vi "11_LaserowaTransmisjaSzeregowaTypuSimplex.vi"() -> ()   [LabVIEW 2017]
uses:
  <vilib>/Instr/_visa.llb/VISA Configure Serial Port (Instr).vi
panel:
  in  "VISA resource name":refnum<visa-resource-name>
  in  "Zakończ":bool
  in  "Wyślij":bool
  in  "Tekst do wysłania":string
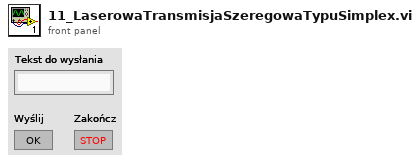
[diagram p1: front panel]
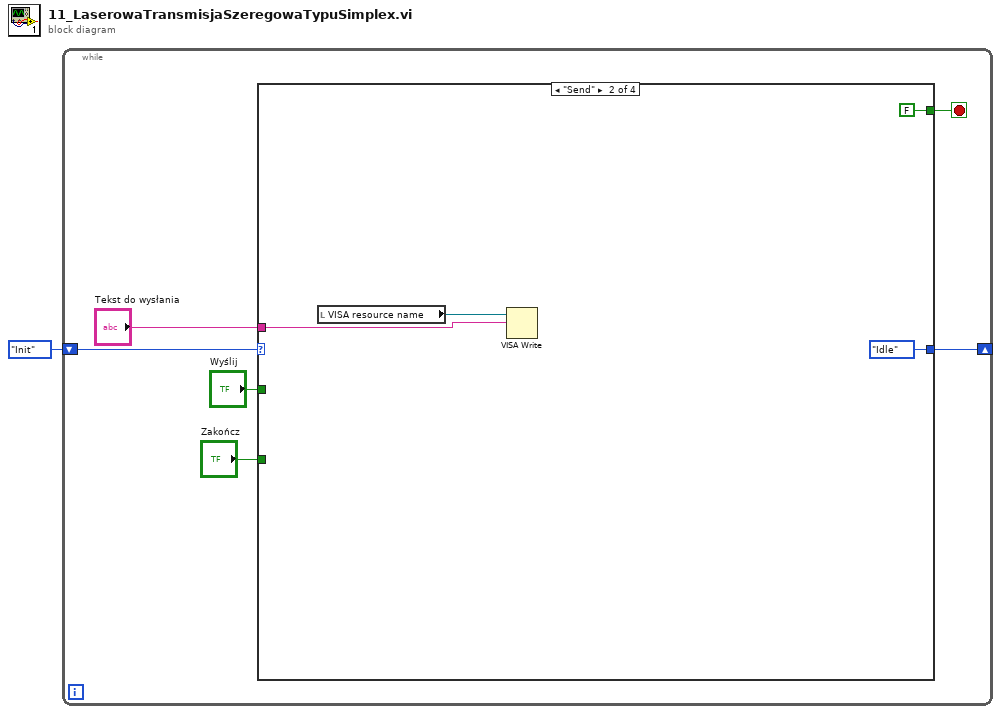
[diagram p0: block diagram]
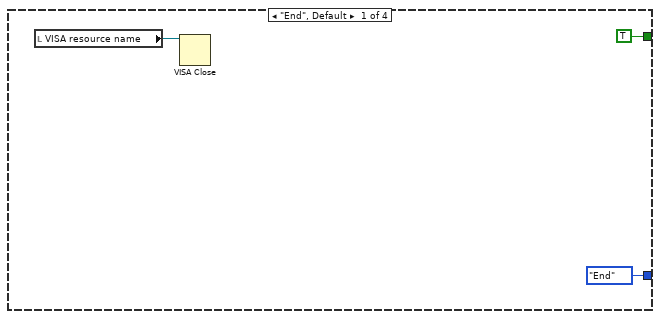
[diagram p2: hidden frame]
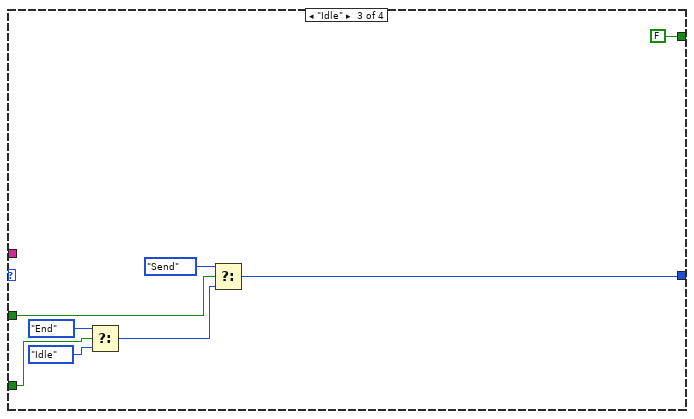
[diagram p3: hidden frame]
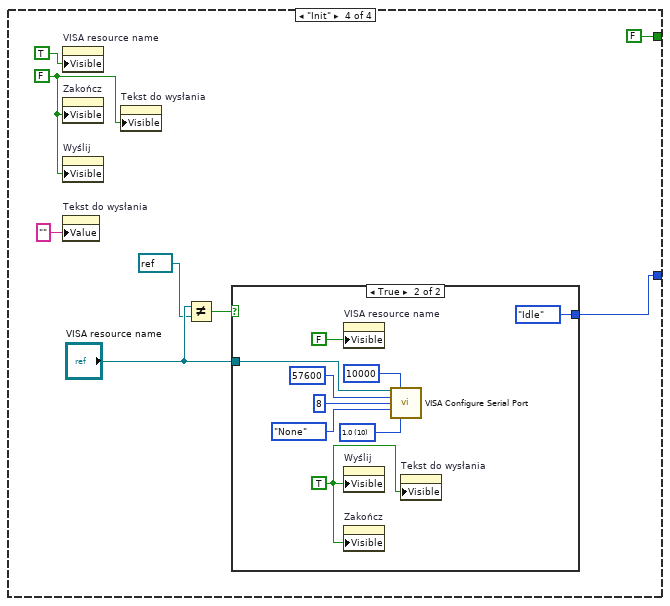
[diagram p4: hidden frame]
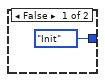
[diagram p5: hidden frame]
diagram:
  n1 = while {
    shift-right: [w3] -> _
    shift-left: enum16{"End", "Send", "Idle", "Init"}."Init" -> [w7]
    stop <- w6 stop-if-true
    n2 = case shown="\"Send\"" w7 {
      tunnel: [TRUE FALSE FALSE FALSE] -> w6
      tunnel: "Zakończ" -> [_ _ w22 _]
      tunnel: "Wyślij" -> [_ _ w19 _]
      tunnel: [enum16{"End", "Send", "Idle", "Init"}."End" enum16{"End", "Send", "Idle", "Init"}."Idle" w16 w29] -> w3
      tunnel: "Tekst do wysłania" -> [_ w11 _ _]
      frame "End", Default {
        n3 = local read "VISA resource name"() -> (w8:refnum<visa-resource-name>)
        n4 = VISA Close(VISA resource name=w8) -> ()  [unwired: 1 in, 1 out]
      }
      frame "Send" {
        n5 = local read "VISA resource name"() -> (w12:refnum<visa-resource-name>)
        n6 = VISA Write(VISA resource name=w12, write buffer=w11) -> ()  [unwired: 1 in, 3 out]
      }
      frame "Idle" {
        n7 = Select(t=enum16{"End", "Send", "Idle", "Init"}."End", s=w22, f=enum16{"End", "Send", "Idle", "Init"}."Idle") -> (s? t:f=w18:enum16{"End", "Send", "Idle", "Init"})
        n8 = Select(t=enum16{"End", "Send", "Idle", "Init"}."Send", s=w19, f=w18) -> (s? t:f=w16:enum16{"End", "Send", "Idle", "Init"})
      }
      frame "Init" {
        w26 = FALSE ("Visible")
        n9 = property on="VISA resource name" class="VISAName"("Visible"=TRUE) -> ()  [unwired: 2 in, 2 out]
        n10 = property on="Zakończ" class="Bool"("Visible"=w26) -> ()  [unwired: 2 in, 2 out]
        n11 = property on="Wyślij" class="Bool"("Visible"=w26) -> ()  [unwired: 2 in, 2 out]
        n12 = property on="Tekst do wysłania" class="Str"("Value"="" ("Tekst do wysłania")) -> ()  [unwired: 2 in, 2 out]
        n13 = property on="Tekst do wysłania" class="Str"("Visible"=w26) -> ()  [unwired: 2 in, 2 out]
        n14 = Not Equal?(x="VISA resource name", y=refnum<visa-resource-name> refnum) -> (x != y?=w28:bool)
        n15 = case shown="True" w28 {
          tunnel: [enum16{"End", "Send", "Idle", "Init"}."Init" enum16{"End", "Send", "Idle", "Init"}."Idle"] -> w29
          tunnel: "VISA resource name" -> [_ w34]
          frame False {
          }
          frame True {
            w32 = TRUE ("Visible")
            w36 = u16 10 items=["1.0"=10, "1.5"=15, "2.0"=20] ("stop bits (10: 1 bit)")
            n16 = property on="VISA resource name" class="VISAName"("Visible"=FALSE) -> ()  [unwired: 2 in, 2 out]
            n17 = property on="Wyślij" class="Bool"("Visible"=w32) -> ()  [unwired: 2 in, 2 out]
            n18 = property on="Zakończ" class="Bool"("Visible"=w32) -> ()  [unwired: 2 in, 2 out]
            n19 = call-poly "VISA Configure Serial Port"("VISA resource name"=w34, "timeout (10sec)"=u32 10000, "baud rate (9600)"=u32 57600, "data bits (8)"=u16 8, "parity (0:none)"=enum16{"None", "Odd", "Even", "Mark", "Space"}."None", "stop bits (10: 1 bit)"=w36) -> ()  [unwired: 8 in, 2 out]
            n20 = property on="Tekst do wysłania" class="Str"("Visible"=w32) -> ()  [unwired: 2 in, 2 out]
          }
        }
      }
    }
  }
